vi "Write Sender.vi"(10 "Sender":refnum<class "Sender.lvclass">, 11 "TEMPLATE Msg in":refnum<class "TEMPLATE Msg.lvclass">) -> (3 "TEMPLATE Msg out":refnum<class "TEMPLATE Msg.lvclass">)   [LabVIEW 2025, in "_Template.lvlib" / "Templates.lvlib" / "TEMPLATE Msg.lvlib" / "TEMPLATE Msg.lvclass"]
uses:
  TEMPLATE Msg.lvclass
  jettl/jettl/Sender/Sender/Sender.lvclass
  TEMPLATE Msg.lvclass/TEMPLATE Msg.ctl
panel:
  # "This front panel should not be manipulated."
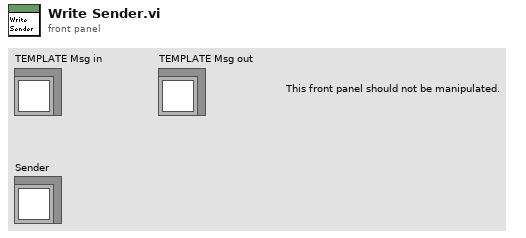
[diagram p1: front panel]
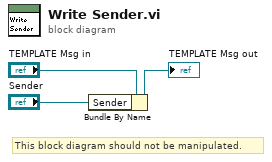
[diagram p0: block diagram]
diagram:
  # "This block diagram should not be manipulated."
  n1 = Bundle By Name(cluster="TEMPLATE Msg in", "Sender"="Sender") -> (→"TEMPLATE Msg out":refnum<class "TEMPLATE Msg.lvclass">)
